vi "Test for OOB Services.vi"(8 "error in":errorcluster, 11 "address":string) -> (0 "error out":errorcluster, 3 "Found OOB Server":bool)   [LabVIEW 2025]
uses:
  reflection_client/RPC Messages/grpc_reflection_v1alpha_ServerReflectionRequest.ctl
  reflection_client/RPC Messages/grpc_reflection_v1alpha_ServerReflectionRequest_message_request/grpc_reflection_v1alpha_ServerReflectionRequest_message_request.lvclass
  reflection_client/RPC Messages/grpc_reflection_v1alpha_ServerReflectionRequest_message_request/grpc_reflection_v1alpha_ServerReflectionRequest_message_request.lvclass/grpc_reflection_v1alpha_ServerReflectionRequest_message_request.ctl
  reflection_client/RPC Messages/grpc_reflection_v1alpha_ServerReflectionResponse_message_response/grpc_reflection_v1alpha_ServerReflectionResponse_message_response.lvclass/grpc_reflection_v1alpha_ServerReflectionResponse_message_response.ctl
  reflection_client/reflection_client.lvlib
  reflection_client/RPC Messages/grpc_reflection_v1alpha_ServerReflectionResponse_message_response/grpc_reflection_v1alpha_ServerReflectionResponse_message_response.lvclass
panel:
  out "Success":bool
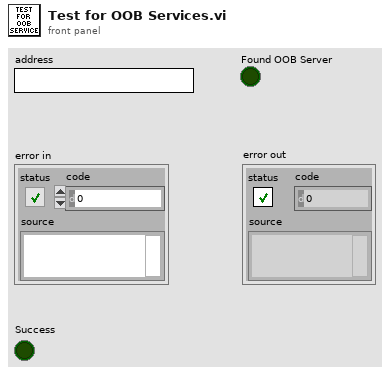
[diagram p1: front panel]
types:
  T1 = typedef "reflection_client.lvlib/grpc_reflection_v1alpha_ServerReflectionRequest.ctl" = cluster{"host":string, "grpc_reflection_v1alpha_ServerReflectionRequest_message_request":refnum<class "grpc_reflection_v1alpha_ServerReflectionRequest_message_request.lvclass">}
  T2 = typedef "grpc-lvsupport-release.lvlib/grpcId.ctl" = u64
  T3 = typedef "reflection_client.lvlib/grpc_reflection_v1alpha_ServerReflectionResponse.ctl" = cluster{"valid_host":string, "original_request":T1, "grpc_reflection_v1alpha_ServerReflectionResponse_message_response":refnum<class "grpc_reflection_v1alpha_ServerReflectionResponse_message_response.lvclass">}
  T4 = typedef "reflection_client.lvlib/grpc_reflection_v1alpha_ListServiceResponse.ctl" = cluster{"service":T5[]}
  T5 = typedef "reflection_client.lvlib/grpc_reflection_v1alpha_ServiceResponse.ctl" = cluster{"name":string}
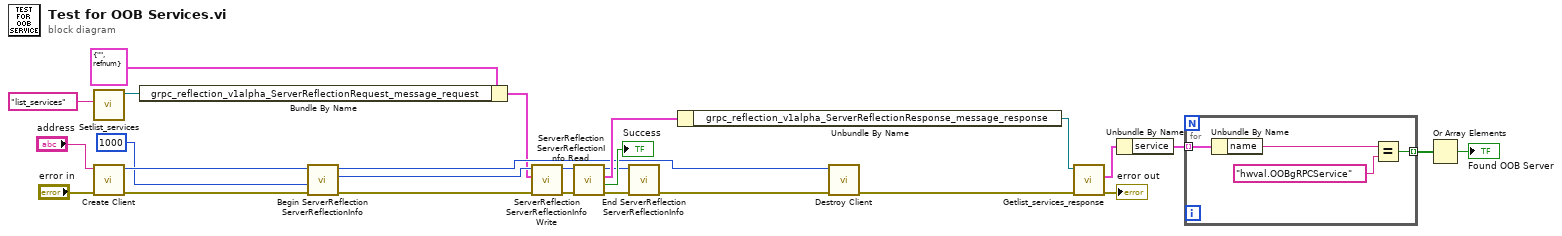
[diagram p0: block diagram]
diagram:
  n1 = call "Setlist_services.vi"("Set_Val"="list_services") -> ("OneOfTemplate out"=w12:refnum<class "grpc_reflection_v1alpha_ServerReflectionRequest_message_request.lvclass">)  [unwired: 9 in, 1 out]
  n2 = call "Create Client.vi"("error in"="error in", "address"="address") -> ("error out"=w23:errorcluster, "gRPC ID Out"=w24:T2)  [unwired: 8 in]
  n3 = Bundle By Name(cluster=T1 {"host"="", "grpc_reflection_v1alpha_ServerReflectionRequest_message_request"=refnum} ("Request Data"), "grpc_reflection_v1alpha_ServerReflectionRequest_message_request"=w12) -> (w8:T1)
  n4 = call "Begin ServerReflection ServerReflectionInfo.vi"("error in"=w23, "timeout (ms)"=1000, "gRPC ID"=w24) -> ("error out"=w15:errorcluster, "Call Id Out"=w16:T2, "gRPC ID out"=w10:T2)  [unwired: 6 in]
  n5 = call "ServerReflection ServerReflectionInfo Write.vi"("error in"=w15, "Request Data"=w8, "Call ID in"=w16) -> ("error out"=w13:errorcluster, "Call ID"=w14:T2)  [unwired: 6 in, 1 out]
  n6 = call "ServerReflection ServerReflectionInfo Read.vi"("error in"=w13, "Call ID in"=w14) -> ("error out"=w7:errorcluster, "Success"=→"Success":bool, "Response Data"=w20:T3, "Call ID"=w5:T2)  [unwired: 6 in]
  n7 = call "End ServerReflection ServerReflectionInfo.vi"("error in"=w7, "Call ID in"=w5) -> ("error out"=w6:errorcluster)  [unwired: 8 in, 1 out]
  n8 = Unbundle By Name(w20) -> ("grpc_reflection_v1alpha_ServerReflectionResponse_message_response"=w19:refnum<class "grpc_reflection_v1alpha_ServerReflectionResponse_message_response.lvclass">)
  n9 = call "Destroy Client.vi"("error in"=w6, "gRPC ID"=w10) -> ("error out"=w17:errorcluster)  [unwired: 9 in]
  n10 = call "Getlist_services_response.vi"("error in (no error)"=w17, "OneOfTemplate in"=w19) -> ("error out"=→"error out":errorcluster, "Get_Val"=w4:T4)  [unwired: 7 in, 1 out]
  n11 = Unbundle By Name(w4) -> ("service"=w3:T5[])
  n12 = for {
    tunnel: w3 -> [w30] mode=indexing
    tunnel: [w27] -> w2 mode=indexing
    n13 = Unbundle By Name(w30) -> ("name"=w29:string)
    n14 = Equal?(x=w29, y="hwval.OOBgRPCService") -> (x = y?=w27:bool)
  }
  n15 = Or Array Elements(Boolean array=w2) -> (logical OR=→"Found OOB Server":bool)
